vi "Auto Loop 0.vi"(2 "Auto State":u8, 3 "Call Context":T1) -> (0 "Loop 0 Data":T2, 1 "SubState 0":T3=enum."driver control")   [LabVIEW 2013]
uses:
  typedefs/State Machine/subStates.ctl
  typedefs/Loop Datatypes/Loop 0 Datatype.ctl
  <vilib>/Rock Robotics/WPI/DriverStation/WPI_DriverStationDerivedRobotMode.ctl
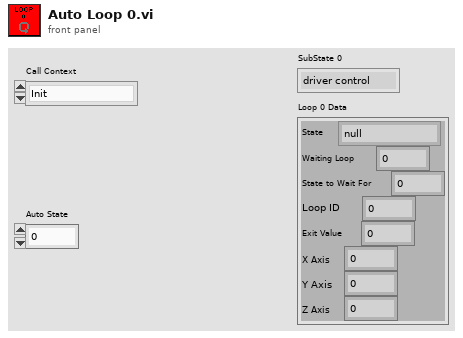
[diagram p1: front panel]
types:
  T1 = typedef "WPI_DriverStationDerivedRobotMode.ctl" = enum16{"Init", "Execute", "Stop"}
  T2 = typedef "Loop 0 Datatype.ctl" = cluster{"State":T3, "Waiting Loop":i32, "State to Wait For":i32, "Loop ID":i32, "Exit Value":i32, "X Axis":dbl, "Y Axis":dbl, "Z Axis":dbl}
  T3 = typedef "subStates.ctl" = enum16{"null", "wait", "driver control", "auto", "manual override", "hold position", "rotate", "pickup", "pass", "recover pass", "load", "goto shoot", "shoot high goal", "shoot low goal", "cancel arm", "cancel shooter", "end", "test"}
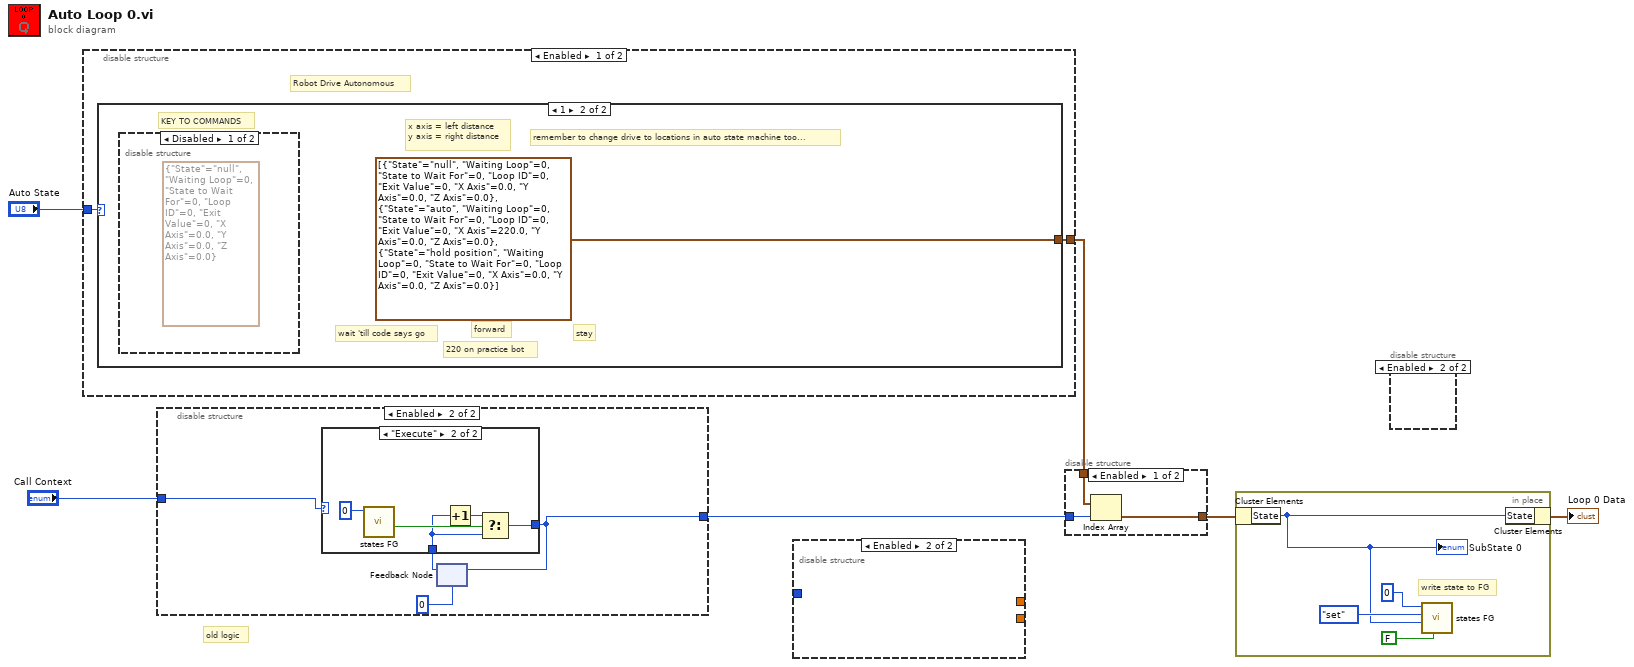
[diagram p0: block diagram]
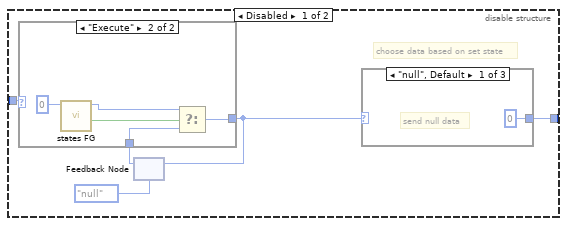
[diagram p2: hidden frame]
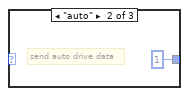
[diagram p3: hidden frame]
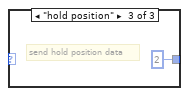
[diagram p4: hidden frame]
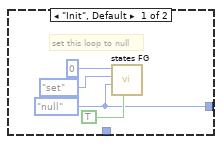
[diagram p5: hidden frame]
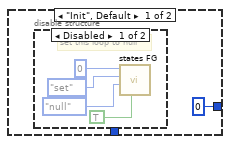
[diagram p6: hidden frame]
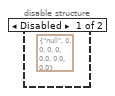
[diagram p8: hidden frame]
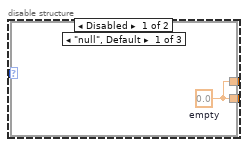
[diagram p9: hidden frame]
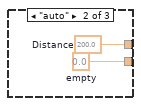
[diagram p10: hidden frame]
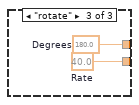
[diagram p11: hidden frame]
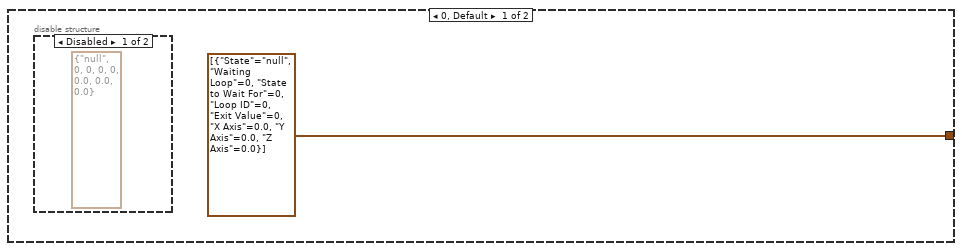
[diagram p13: hidden frame]
diagram:
  # "old logic"
  n1 = disable-structure shown="Enabled" {
    disable-tunnel: "Auto State" -> [w8 _]
    disable-tunnel: [w7 _] -> w4
    frame Enabled {
      # "Robot Drive Autonomous"
      n2 = case shown="1" w8 {
        tunnel: [T2[] [{"State"=enum."null", "Waiting Loop"=0, "State to Wait For"=0, "Loop ID"=0, "Exit Value"=0, "X Axis"=0.0, "Y Axis"=0.0, "Z Axis"=0.0}] T2[] [{"State"=enum."null", "Waiting Loop"=0, "State to Wait For"=0, "Loop ID"=0, "Exit Value"=0, "X Axis"=0.0, "Y Axis"=0.0, "Z Axis"=0.0}, {"State"=enum."auto", "Waiting Loop"=0, "State to Wait For"=0, "Loop ID"=0, "Exit Value"=0, "X Axis"=220.0, "Y Axis"=0.0, "Z Axis"=0.0}, {"State"=enum."hold position", "Waiting Loop"=0, "State to Wait For"=0, "Loop ID"=0, "Exit Value"=0, "X Axis"=0.0, "Y Axis"=0.0, "Z Axis"=0.0}]] -> w7
        frame 0, Default {
          n3 = disable-structure shown="Disabled" {
            frame Disabled {
              (unwired) T2 {"State"=enum."null", "Waiting Loop"=0, "State to Wait For"=0, "Loop ID"=0, "Exit Value"=0, "X Axis"=0.0, "Y Axis"=0.0, "Z Axis"=0.0} ("Loop 0 Data")
            }
            frame Enabled {
            }
          }
        }
        frame 1 {
          # "remember to change drive to locations in auto state machine too..."
          # "220 on practice bot"
          # "x axis = left distance\ny axis = right distance"
          # "wait 'till code says go"
          # "stay"
          # "forward"
          # "KEY TO COMMANDS"
          n4 = disable-structure shown="Disabled" {
            frame Disabled {
              (unwired) T2 {"State"=enum."null", "Waiting Loop"=0, "State to Wait For"=0, "Loop ID"=0, "Exit Value"=0, "X Axis"=0.0, "Y Axis"=0.0, "Z Axis"=0.0} ("Loop 0 Data")
            }
            frame Enabled {
            }
          }
        }
      }
    }
    frame Disabled {
    }
  }
  n5 = disable-structure shown="Enabled" {
    disable-tunnel: "Call Context" -> [w15 w29]
    disable-tunnel: [w11 w28] -> w1
    frame Disabled {
      # "choose data based on set state"
      n6 = feedback #1(subStates."null" ("subState out")) -> (w14:T3)
      n7 = case shown="\"Execute\"" w15 {
        tunnel: w14 -> [_ w24]
        tunnel: [w19 w26] -> w12
        frame "Init", Default {
          w19 = subStates."null" ("subState in")
          # "set this loop to null"
          n8 = call "states FG.vi"("exit in"=TRUE, "subState in"=w19, "menu (get)"=enum16{"set", "get"}."set", "Loop ID"=0) -> ()  [unwired: 4 in, 4 out]
        }
        frame "Execute" {
          n9 = call "states FG.vi"("Loop ID"=0) -> ("exit out"=w25:bool, "subState out"=w23:T3)  [unwired: 7 in, 2 out]
          n10 = Select(t=w23, s=w25, f=w24) -> (s? t:f=w26:T3)
        }
      }
      n11 = feedback-in #1(w12) -> ()
      n12 = case shown="\"null\", Default" w12 {
        tunnel: [0 ("index") 1 ("index") 2 ("index")] -> w11
        frame "null", Default {
          # "send null data"
        }
        frame "auto" {
          # "send auto drive data"
        }
        frame "hold position" {
          # "send hold position data"
        }
      }
    }
    frame Enabled {
      n13 = feedback #2(0) -> (w31:i32)
      n14 = case shown="\"Execute\"" w29 {
        tunnel: w31 -> [_ w38]
        tunnel: [0 ("subState out") w40] -> w28
        frame "Init", Default {
          n15 = disable-structure shown="Disabled" {
            frame Disabled {
              # "set this loop to null"
              n16 = call "states FG.vi"("exit in"=TRUE, "subState in"=subStates."null", "menu (get)"=enum16{"set", "get"}."set", "Loop ID"=0) -> ()  [unwired: 4 in, 4 out]
            }
            frame Enabled {
            }
          }
        }
        frame "Execute" {
          n17 = call "states FG.vi"("Loop ID"=0) -> ("exit out"=w39:bool)  [unwired: 7 in, 3 out]
          n18 = Increment(x=w38) -> (x+1=w37:i32)
          n19 = Select(t=w37, s=w39, f=w38) -> (s? t:f=w40:i32)
        }
      }
      n20 = feedback-in #2(w28) -> ()
    }
  }
  n21 = disable-structure shown="Enabled" {
    disable-tunnel: [w44 _] -> _
    disable-tunnel: _ -> [w43 _]
    disable-tunnel: [w42 _] -> _
    frame Disabled {
      n22 = case shown="\"null\", Default" w43 {
        tunnel: [w45 w47 w49] -> w44
        tunnel: [w45 w46 w48] -> w42
        frame "null", Default {
          w45 = 0.0  # empty
        }
        frame "auto" {
          w46 = 0.0  # empty
          w47 = 200.0  # Distance
        }
        frame "rotate" {
          w48 = 40.0  # Rate
          w49 = 180.0  # Degrees
        }
      }
    }
    frame Enabled {
    }
  }
  n23 = disable-structure shown="Enabled" {
    disable-tunnel: w4 -> [w52 _]
    disable-tunnel: [w51 _] -> w3
    disable-tunnel: w1 -> [w50 _]
    frame Enabled {
      n24 = Index Array(array=w52, index=w50) -> (element=w51:T2)
    }
    frame Disabled {
    }
  }
  n25 = in-place {
    # "write state to FG"
    n26 = in-place-cluster #3(w3) -> ("State"=w53:T3)
    "SubState 0" <- w53
    n27 = call "states FG.vi"("exit in"=FALSE, "subState in"=w53, "menu (get)"=enum16{"set", "get"}."set", "Loop ID"=0) -> ()  [unwired: 4 in, 4 out]
    n28 = in-place-cluster #3("State"=w53) -> (→"Loop 0 Data":T2)
  }
  n29 = disable-structure shown="Enabled" {
    frame Disabled {
      (unwired) T2 {"State"=enum."null", "Waiting Loop"=0, "State to Wait For"=0, "Loop ID"=0, "Exit Value"=0, "X Axis"=0.0, "Y Axis"=0.0, "Z Axis"=0.0} ("Loop 0 Data 2")
    }
    frame Enabled {
    }
  }
